vi "PCO_GetHWIOSignalDescriptor.vi"(8 "error in (no error)":errorcluster {"code" format="%x"}, 10 "wSignalNum":u16, 11 "ph":u64) -> (0 "error out":errorcluster {"code" format="%x"}, 1 "strSignalDesc":T1, 2 "ErrorMessage":i32 format="%x", 3 "ph out":u64)   [LabVIEW 2019, in "SDK.lvlib" / "TimingControl.lvlib"]
doc: "<b>Description:</b>\nThis function does retrieve the description of a distinct hardware I/O signal line. The number of available hardware I/O signal lines can be queried with PCO_GetHWIOSignalCount.\nOnly predefined signals can be routed to distinct signal lines. With the values returned in the PCO_Single_Signal_Desc structure available options for each I/O signal line can be determined. With these options in mind the PCO Signal structure for the call to PCO_SetHWIOSignal can be prepared.\nOptional parameters can be set for some of the predefined signals, allowing better control of the signal. Optional Parameters are available, when one of the SIGNAL_DEF_PARAM bits is set in the Signal Definitions Bits. Descriptions for the additional parameters can be found in the appropriate listing, which is defined through the Signal Functionality returned from the PCO_GetHWIOSignal function.\nAdditional information about input / output lines can be found in the respective camera manual.\n\n<b>Supported camera type:</b>\npco.edge, pco.dimax\n\n<b>Descriptor dependency:</b>\ndwGeneralCapsDESC1: HW_IO_SIGNAL_DESCRIPTOR"
uses:
  TimingControl.lvlib
  Structures/Structures.lvlib
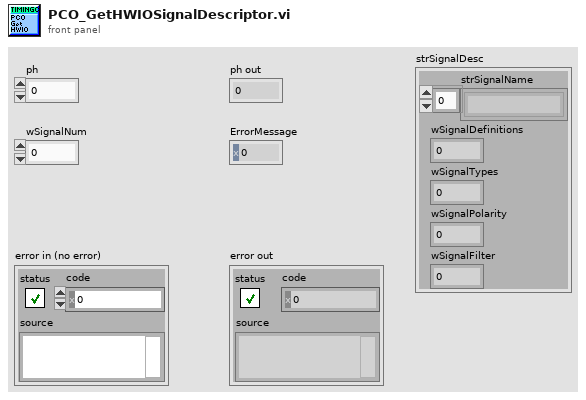
[diagram p1: front panel]
types:
  T1 = cluster{"strSignalName":string[], "wSignalDefinitions":u16, "wSignalTypes":u16, "wSignalPolarity":u16, "wSignalFilter":u16}
  T2 = cluster{"wSize":u16, "ZZwAlignDummy1":u16, "strSignalName":cluster{cluster{u8, u8, u8, u8, u8, u8, u8, u8, u8, u8, u8, u8, u8, u8, u8, u8, u8, u8, u8, u8, u8, u8, u8, u8, u8}, cluster{u8, u8, u8, u8, u8, u8, u8, u8, u8, u8, u8, u8, u8, u8, u8, u8, u8, u8, u8, u8, u8, u8, u8, u8, u8}, cluster{u8, u8, u8, u8, u8, u8, u8, u8, u8, u8, u8, u8, u8, u8, u8, u8, u8, u8, u8, u8, u8, u8, u8, u8, u8}, cluster{u8, u8, u8, u8, u8, u8, u8, u8, u8, u8, u8, u8, u8, u8, u8, u8, u8, u8, u8, u8, u8, u8, u8, u8, u8}}, "wSignalDefinitions":u16, "wSignalTypes":u16, "wSignalPolarity":u16, "wSignalFilter":u16, "dwDummy":cluster{u32, u32, u32, u32, u32, u32, u32, u32, u32, u32, u32, u32, u32, u32, u32, u32, u32, u32, u32, u32, u32, u32}}
  T3 = cluster{cluster{u8, u8, u8, u8, u8, u8, u8, u8, u8, u8, u8, u8, u8, u8, u8, u8, u8, u8, u8, u8, u8, u8, u8, u8, u8}, cluster{u8, u8, u8, u8, u8, u8, u8, u8, u8, u8, u8, u8, u8, u8, u8, u8, u8, u8, u8, u8, u8, u8, u8, u8, u8}, cluster{u8, u8, u8, u8, u8, u8, u8, u8, u8, u8, u8, u8, u8, u8, u8, u8, u8, u8, u8, u8, u8, u8, u8, u8, u8}, cluster{u8, u8, u8, u8, u8, u8, u8, u8, u8, u8, u8, u8, u8, u8, u8, u8, u8, u8, u8, u8, u8, u8, u8, u8, u8}}
  T4 = cluster{u8, u8, u8, u8, u8, u8, u8, u8, u8, u8, u8, u8, u8, u8, u8, u8, u8, u8, u8, u8, u8, u8, u8, u8, u8}[]
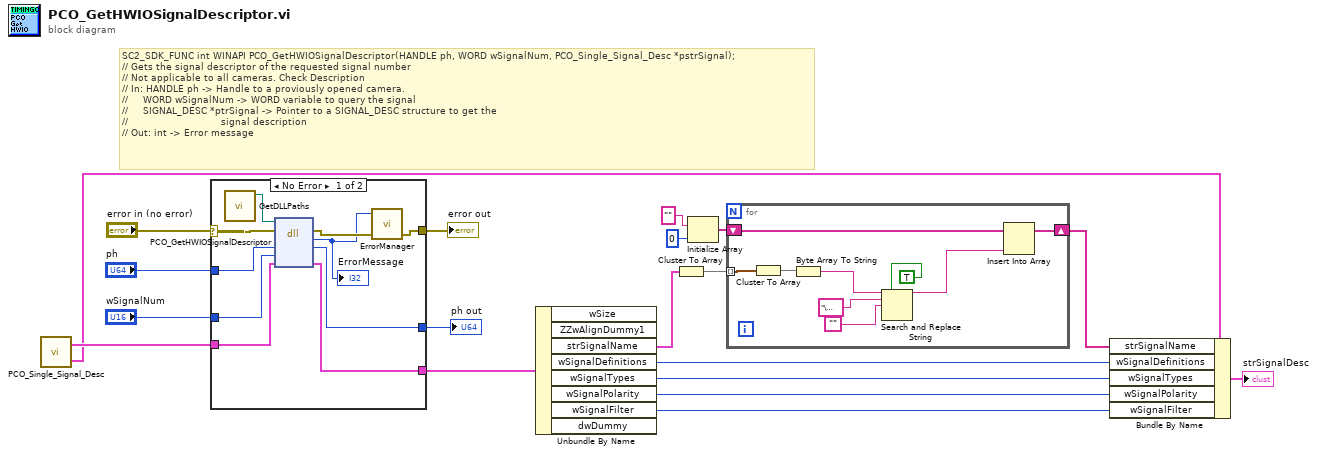
[diagram p0: block diagram]
diagram:
  # "SC2_SDK_FUNC int WINAPI PCO_GetHWIOSignalDescriptor(HANDLE ph, WORD wSignalNum, PCO_Single_Signal_Desc *pstrSignal);\n// Gets the signal descriptor of the requested signal number\n// Not applicable to all cameras. Check Description\n// In: HANDLE ph -> Handle to a proviously opened camera.\n//     WORD wSignalNum -> WORD variable to query the signal\n//     SIGNAL_DESC *ptrSignal -> Pointer to a SIGNAL_DESC structure to get the\n//                               signal description\n// Out: int -> Error message"
  n1 = call "PCO_Single_Signal_Desc.vi"() -> ("PCO_Single_Signal_Desc"=w12:T1, "PCO_Single_Signal_Desc_Raw"=w15:T2)  [unwired: 4 in, 2 out]
  n2 = case shown="No Error" "error in (no error)" {
    selector: "error in (no error)" -> [w22 w32]
    tunnel: "ph" -> [w29 w31]
    tunnel: [w28 w31] -> w18
    tunnel: "wSignalNum" -> [w27 _]
    tunnel: [w24 w32] -> w16
    tunnel: w15 -> [w26 w30]
    tunnel: [w21 w30] -> w13
    frame No Error {
      n3 = call "GetDLLPaths.vi"() -> ("SC2_Cam_Path"=w20:path)  [unwired: 8 in, 3 out]
      n4 = dll-call lib="?" fn="PCO_GetHWIOSignalDescriptor"(path in=w20, error in=w22, "ph"=w29, "wSignalNum"=w27, "pstrSignal"=w26) -> (error out=w25:errorcluster, "return type"=w23:i32, "ph"=w28:u64, "pstrSignal"=w21:T2)  [unwired: 2 in, 1 out]
      "ErrorMessage" <- w23
      n5 = call "ErrorManager.vi"("error in (no error)"=w25, "error code"=w23) -> ("error out"=w24:errorcluster)  [unwired: 2 in, 1 out]
    }
    frame Error {
    }
  }
  "ph out" <- w18
  "error out" <- w16
  n6 = Unbundle By Name(w13) -> ("strSignalName"=w7:T3, "wSignalDefinitions"=w5:u16, "wSignalTypes"=w4:u16, "wSignalPolarity"=w3:u16, "wSignalFilter"=w2:u16)  [unwired: 3 out]
  n7 = Cluster To Array(cluster=w7) -> (array=w8:T4)
  n8 = Initialize Array("", 0 ("dimension size")) -> (w9:string[])
  n9 = for {
    shift-right: [w40] -> w6
    shift-left: w9 -> [w41]
    tunnel: w8 -> [w33] mode=indexing
    n10 = Cluster To Array(cluster=w33) -> (array=w35:u8[])
    n11 = Byte Array To String(unsigned byte array=w35) -> (string=w39:string)
    n12 = Search and Replace String(replace all?=TRUE ("replace all? (F)"), input string=w39, search string="\u0000", replace string="" ("replace string (\"\")")) -> (result string=w34:string)  [unwired: 4 in, 3 out]
    n13 = Insert Into Array(array=w41, new element=w34) -> (w40:string[])  [unwired: 1 in]
  }
  n14 = Bundle By Name(cluster=w12, "strSignalName"=w6, "wSignalDefinitions"=w5, "wSignalTypes"=w4, "wSignalPolarity"=w3, "wSignalFilter"=w2) -> (→"strSignalDesc":T1)
